vi "unpack_si.vi"(11 "payload":u64) -> (0 "right_hand":T1(array[cluster]), 1 "left_hand":T1(array[cluster]), 2 "eye_ray":sgl[](array[numeric]), 3 "head_pose":sgl[](array[numeric]), 4 "error":bool, 5 "valid":u32)   [LabVIEW 2023]
panel:
  in  "si_hand_joint":T2
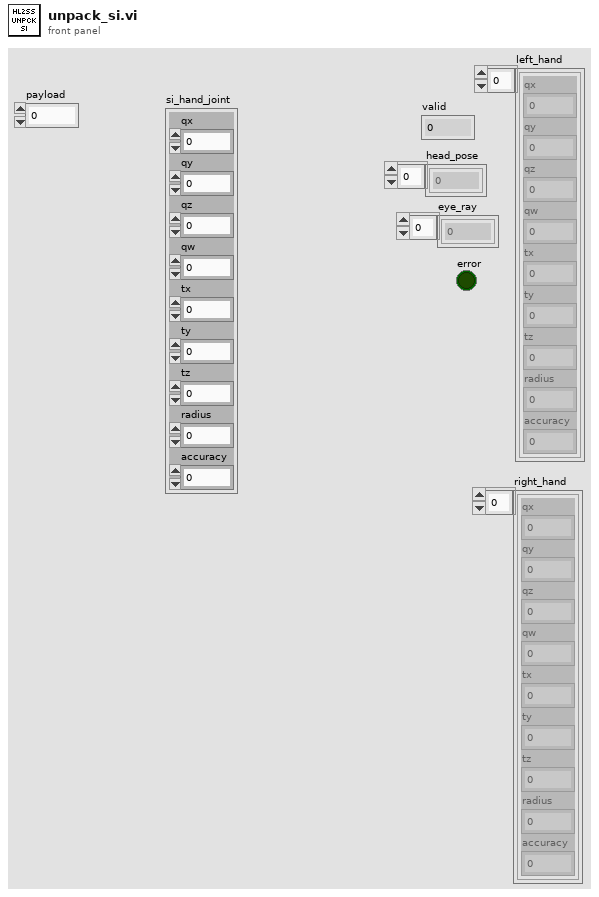
[diagram p1: front panel]
types:
  T1 = cluster{"qx":sgl, "qy":sgl, "qz":sgl, "qw":sgl, "tx":sgl, "ty":sgl, "tz":sgl, "radius":sgl, "accuracy":i32}[]
  T2 = cluster{"qx":sgl, "qy":sgl, "qz":sgl, "qw":sgl, "tx":sgl, "ty":sgl, "tz":sgl, "radius":sgl, "accuracy":i32}
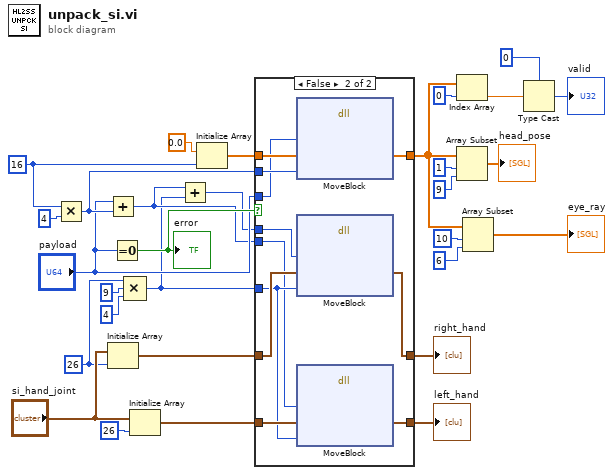
[diagram p0: block diagram]
diagram:
  w20 = 16 ("dimension size")
  w25 = 26 ("dimension size")
  n1 = Multiply(x=w20, y=4) -> (x*y=w18:i32)
  n2 = Add(x="payload", y=w18) -> (x+y=w16:u64)
  n3 = Initialize Array("si_hand_joint", w25) -> (w26:T1)
  n4 = Equal To 0?(x="payload") -> (x = 0?=w30:bool)
  "error" <- w30
  n5 = Compound Arithmetic op=MULTIPLY(w25, 9 ("value"), 4 ("value")) -> (w15:i32)
  n6 = Initialize Array("si_hand_joint", 26 ("dimension size")) -> (w29:T1)
  n7 = Add(x=w16, y=w15) -> (x+y=w14:u64)
  n8 = Initialize Array(sgl 0.0 ("element"), w20) -> (w21:sgl[])
  n9 = case shown="False" w30 {
    tunnel: "payload" -> [_ w37]
    tunnel: w29 -> [w33 w43]
    tunnel: [w33 w44] -> w2
    tunnel: w26 -> [w32 w42]
    tunnel: w15 -> [_ w40]
    tunnel: [w32 w41] -> w1
    tunnel: w21 -> [w31 w39]
    tunnel: w18 -> [_ w38]
    tunnel: w16 -> [_ w36]
    tunnel: w14 -> [_ w35]
    tunnel: [w31 w34] -> w7
    frame True {
    }
    frame False {
      n10 = dll-call lib="LabVIEW" fn="MoveBlock"("ps"=w37, "pd"=w39, "size"=w38) -> ("pd"=w34:sgl[])  [unwired: 6 in, 2 out]
      n11 = dll-call lib="LabVIEW" fn="MoveBlock"("ps"=w35, "pd"=w42, "size"=w40) -> ("pd"=w41:T1)  [unwired: 6 in, 2 out]
      n12 = dll-call lib="LabVIEW" fn="MoveBlock"("ps"=w36, "pd"=w43, "size"=w40) -> ("pd"=w44:T1)  [unwired: 6 in, 2 out]
    }
  }
  "left_hand" <- w2
  "right_hand" <- w1
  n13 = Index Array(array=w7, index=0) -> (element=w4:sgl)
  n14 = Array Subset(array=w7, index=1, length=9) -> (→"head_pose":sgl[])
  n15 = Array Subset(array=w7, index=10, length=6) -> (→"eye_ray":sgl[])
  n16 = Type Cast(type=u32 0 ("index"), x=w4) -> (*(type *) &x=→"valid":u32)
